vi "boot.vi"   [LabVIEW 2016]
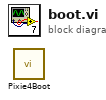
[diagram p0: block diagram]
diagram:
  n1 = call "Pixie4Boot.vi"() -> ()  [unwired: 11 in, 1 out]
